vi "ObserverDemo.vi"() -> ()   [LabVIEW 2017]
uses:
  ForecastDisplay/ForecastDisplay.lvclass
  C:/Users/fflores/Documents/LabVIEW-Open-Projects/LabIVEW OOP Design Patterns/Observer Pattern/Observer Pattern Example/Observer/Observer.lvclass
  Weather Station/WeatherData.lvclass
  General Display/GeneralDisplay.lvclass
  StatisticsDisplay/StatisticsDisplay.lvclass
panel:
  in  "Stop Button":bool
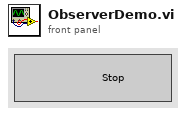
[diagram p1: front panel]
types:
  T1 = cluster{"Temperature":dbl, "Humidity":dbl, "Pressure":dbl}
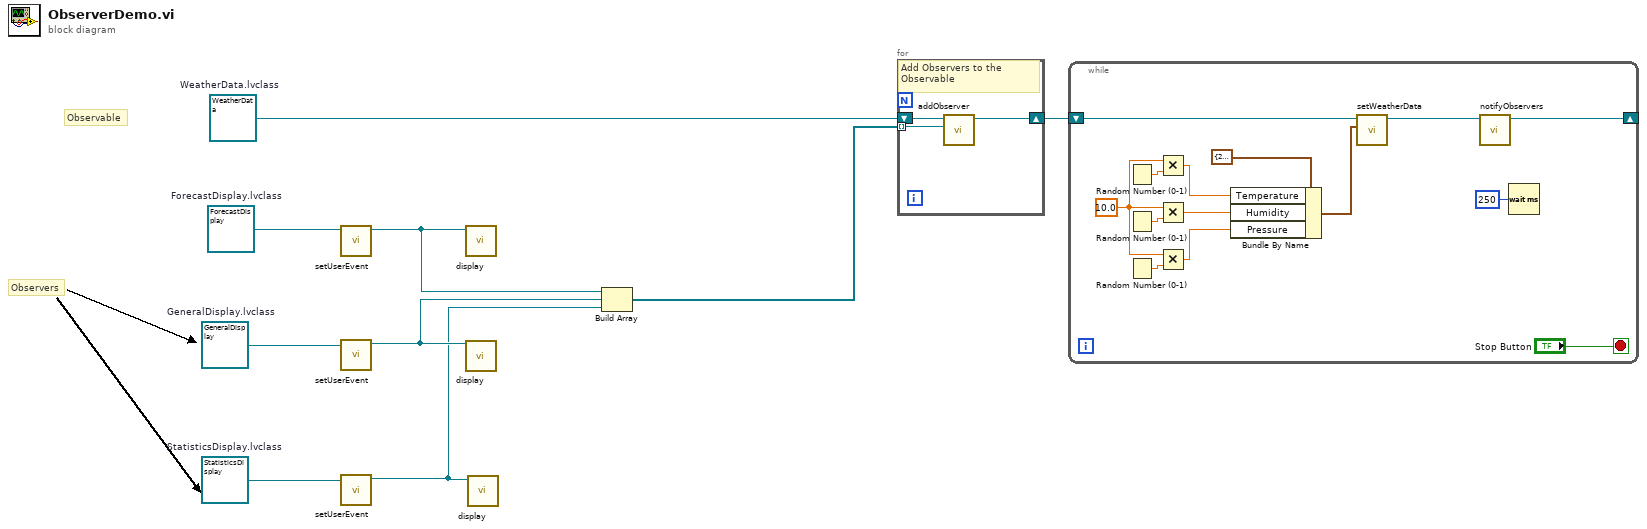
[diagram p0: block diagram]
diagram:
  w1 = refnum<class "StatisticsDisplay.lvclass"> refnum  # StatisticsDisplay.lvclass
  w6 = refnum<class "GeneralDisplay.lvclass"> refnum  # GeneralDisplay.lvclass
  w8 = refnum<class "WeatherData.lvclass"> refnum  # WeatherData.lvclass
  w9 = refnum<class "ForecastDisplay.lvclass"> refnum  # ForecastDisplay.lvclass
  # "Observers"
  # "Observable"
  n1 = call-dynamic "setUserEvent.vi"("ForecastDisplay in"=w9) -> ("ForecastDisplay out"=w5:refnum<class "ForecastDisplay.lvclass">)  [unwired: 9 in, 1 out]
  n2 = call-dynamic "setUserEvent.vi"("GeneralDisplay in"=w6) -> ("GeneralDisplay out"=w4:refnum<class "GeneralDisplay.lvclass">)  [unwired: 9 in, 1 out]
  n3 = call-dynamic "setUserEvent.vi"("StatisticsDisplay in"=w1) -> ("StatisticsDisplay out"=w2:refnum<class "StatisticsDisplay.lvclass">)  [unwired: 9 in, 1 out]
  n4 = call-dynamic "display.vi"("ForecastDisplay in"=w5) -> ()  [unwired: 9 in, 2 out]
  n5 = call-dynamic "display.vi"("GeneralDisplay in"=w4) -> ()  [unwired: 9 in, 2 out]
  n6 = call-dynamic "display.vi"("StatisticsDisplay in"=w2) -> ()  [unwired: 9 in, 2 out]
  n7 = Build Array(w5, w4, w2) -> (w3:refnum<class "Observer.lvclass">[])
  n8 = for {
    tunnel: w3 -> [w10] mode=indexing
    shift-right: [w11] -> w7
    shift-left: w8 -> [w12]
    # "Add Observers to the Observable"
    n9 = call-dynamic "addObserver.vi"("Observer.lvclass"=w10, "Observable in"=w12) -> ("Observable out"=w11:refnum<class "WeatherData.lvclass">)  [unwired: 8 in, 1 out]
  }
  n10 = while {
    shift-right: [w13] -> _
    shift-left: w7 -> [w26]
    stop <- "Stop Button" stop-if-true
    w16 = 10.0
    n11 = Random Number (0-1)() -> (number: 0 to 1=w23:dbl)
    n12 = Random Number (0-1)() -> (number: 0 to 1=w22:dbl)
    n13 = Random Number (0-1)() -> (number: 0 to 1=w21:dbl)
    n14 = Multiply(x=w16, y=w23) -> (x*y=w19:dbl)
    n15 = Multiply(x=w16, y=w22) -> (x*y=w18:dbl)
    n16 = Multiply(x=w16, y=w21) -> (x*y=w17:dbl)
    n17 = Bundle By Name(cluster=T1 {"Temperature"=20.0, "Humidity"=15.0, "Pressure"=25.0} ("WeatherData"), "Temperature"=w19, "Humidity"=w18, "Pressure"=w17) -> (w24:T1)
    n18 = call-dynamic "setWeatherData.vi"("WeatherData"=w24, "WeatherData in"=w26) -> ("WeatherData out"=w20:refnum<class "WeatherData.lvclass">)  [unwired: 8 in, 1 out]
    n19 = call-dynamic "notifyObservers.vi"("WeatherData in"=w20) -> ("WeatherData out"=w13:refnum<class "WeatherData.lvclass">)  [unwired: 9 in, 1 out]
    n20 = Wait (ms)(milliseconds to wait=u32 250) -> ()  [unwired: 1 out]
  }
